vi "Main.vi"(7 "sweep rate, /min":dbl=0.2, 8 "sweep to:":dbl=4.0, 9 "sweep":T8(radio)=enum."2636a_smub") -> ()   [LabVIEW 2021] (continued)
                    n4073 = Number To Decimal String(number=w5385) -> (decimal integer string=w5387:string)  [unwired: 1 in]
                    n4074 = GPIB Write(0:w5387, 1:w5389, 2:i16 1 ("mode (0)")) -> ()  [unwired: 2 in, 2 out]
                  }
                  frame "2636_smua_step" {
                    # "sweep voltage on 2636a smua"
                    n4075 = property on="Step Channel" class="DigNum (strict)"() -> ("Value"=w5395:dbl)  [unwired: 2 in, 2 out]
                    n4076 = property on="Mini steps" class="DigNum (strict)"() -> ("Value"=w5393:dbl)  [unwired: 2 in, 2 out]
                    n4077 = property on="2614A_addr_step" class="VISAName"() -> ("Value"=w5394:refnum<visa-resource-name>)  [unwired: 2 in, 2 out]
                    n4078 = Subtract(x=w5392, y=w5395) -> (x-y=w5396:dbl)
                    n4079 = Divide(x=w5396, y=w5393) -> (x/y=w5397:dbl)
                    n4080 = for {
                      N: w5393 -> [_]
                      tunnel: w5395 -> [w5411]
                      tunnel: w5397 -> [w5410]
                      tunnel: w5394 -> [w5407]
                      i -> [w5406]
                      n4081 = Increment(x=w5406) -> (x+1=w5405:i32)
                      n4082 = Multiply(x=w5410, y=w5405) -> (x*y=w5409:dbl)
                      n4083 = Add(x=w5409, y=w5411) -> (x+y=w5403:dbl)
                      n4084 = property on="Lead Chanl_step" class="Enum (strict)"() -> ("Value"=w5402:T4)  [unwired: 2 in, 2 out]
                      n4085 = property on="step" class="RadioBtnsControl (strict)"() -> ("Value"=w5401:T5)  [unwired: 2 in, 2 out]
                      n4086 = call "setLevel.vi"("VISA resource name 2"=w5407, "Source"=Source."Voltage", "Channel"=Channel."a", "SourceLevel"=w5403) -> ("VISA resource name"=w5404:refnum<visa-resource-name>)  [unwired: 1 in, 2 out]
                      n4087 = property on="diagonal step" class="Bool (strict)"() -> ("Value"=w5400:bool)  [unwired: 2 in, 2 out]
                      n4088 = Wait (ms)(milliseconds to wait=u32 12) -> ()  [unwired: 1 out]
                      n4089 = Equal?(x=w5402, y=w5401) -> (x = y?=w5399:bool)
                      n4090 = property on="Current Step Value" class="DigNum (strict)"("Value"=w5403) -> ()  [unwired: 2 in, 2 out]
                      n4091 = And(x=w5400, y=w5399) -> (x .and. y?=w5398:bool)
                      n4092 = case shown="True" w5398 {
                        tunnel: w5403 -> [_ w5421]
                        tunnel: w5404 -> [_ w5416]
                        frame False {
                        }
                        frame True {
                          n4093 = property on="Step Slope" class="DigNum (strict)"() -> ("Value"=w5415:dbl)  [unwired: 2 in, 2 out]
                          n4094 = property on="Step Offset" class="DigNum (strict)"() -> ("Value"=w5414:dbl)  [unwired: 2 in, 2 out]
                          n4095 = Multiply(x=w5421, y=w5415) -> (x*y=w5420:dbl)
                          n4096 = Add(x=w5420, y=w5414) -> (x+y=w5417:dbl)
                          n4097 = call "setLevel.vi"("VISA resource name 2"=w5416, "Source"=Source."Voltage", "Channel"=Channel."b", "SourceLevel"=w5417) -> ()  [unwired: 1 in, 3 out]
                        }
                      }
                    }
                  }
                  frame "2636_smub_step" {
                    # "sweep voltage on 2636a smua"
                    n4098 = property on="Step Channel" class="DigNum (strict)"() -> ("Value"=w5425:dbl)  [unwired: 2 in, 2 out]
                    n4099 = property on="Mini steps" class="DigNum (strict)"() -> ("Value"=w5423:dbl)  [unwired: 2 in, 2 out]
                    n4100 = property on="2614A_addr_step" class="VISAName"() -> ("Value"=w5424:refnum<visa-resource-name>)  [unwired: 2 in, 2 out]
                    n4101 = Subtract(x=w5422, y=w5425) -> (x-y=w5426:dbl)
                    n4102 = Divide(x=w5426, y=w5423) -> (x/y=w5427:dbl)
                    n4103 = for {
                      N: w5423 -> [_]
                      tunnel: w5425 -> [w5441]
                      tunnel: w5427 -> [w5440]
                      tunnel: w5424 -> [w5437]
                      i -> [w5436]
                      n4104 = Increment(x=w5436) -> (x+1=w5435:i32)
                      n4105 = Multiply(x=w5440, y=w5435) -> (x*y=w5439:dbl)
                      n4106 = Add(x=w5439, y=w5441) -> (x+y=w5433:dbl)
                      n4107 = property on="Lead Chanl_step" class="Enum (strict)"() -> ("Value"=w5432:T4)  [unwired: 2 in, 2 out]
                      n4108 = property on="step" class="RadioBtnsControl (strict)"() -> ("Value"=w5431:T5)  [unwired: 2 in, 2 out]
                      n4109 = call "setLevel.vi"("VISA resource name 2"=w5437, "Source"=Source."Voltage", "Channel"=Channel."b", "SourceLevel"=w5433) -> ("VISA resource name"=w5434:refnum<visa-resource-name>)  [unwired: 1 in, 2 out]
                      n4110 = property on="diagonal step" class="Bool (strict)"() -> ("Value"=w5430:bool)  [unwired: 2 in, 2 out]
                      n4111 = Wait (ms)(milliseconds to wait=u32 12) -> ()  [unwired: 1 out]
                      n4112 = Equal?(x=w5432, y=w5431) -> (x = y?=w5429:bool)
                      n4113 = And(x=w5430, y=w5429) -> (x .and. y?=w5428:bool)
                      n4114 = property on="Current Step Value" class="DigNum (strict)"("Value"=w5433) -> ()  [unwired: 2 in, 2 out]
                      n4115 = case shown="True" w5428 {
                        tunnel: w5433 -> [_ w5451]
                        tunnel: w5434 -> [_ w5446]
                        frame False {
                        }
                        frame True {
                          n4116 = property on="Step Slope" class="DigNum (strict)"() -> ("Value"=w5445:dbl)  [unwired: 2 in, 2 out]
                          n4117 = property on="Step Offset" class="DigNum (strict)"() -> ("Value"=w5444:dbl)  [unwired: 2 in, 2 out]
                          n4118 = Multiply(x=w5451, y=w5445) -> (x*y=w5450:dbl)
                          n4119 = Add(x=w5450, y=w5444) -> (x+y=w5447:dbl)
                          n4120 = call "setLevel.vi"("VISA resource name 2"=w5446, "Source"=Source."Voltage", "Channel"=Channel."a", "SourceLevel"=w5447) -> ()  [unwired: 1 in, 3 out]
                        }
                      }
                    }
                  }
                  frame "time_step", Default {
                    # "do not sweep, just time"
                  }
                  frame "iPS_step" {
                    # "step magnetic field"
                    n4121 = stacked-sequence {
                      tunnel: w5452 -> [w5453 w5466 _]
                      frame #0 {
                        n4122 = property on="Table Index" class="DigNum (strict)"() -> ("Value"=w5456:dbl)  [unwired: 2 in, 2 out]
                        n4123 = Equal?(x=w5456, y=0.0) -> (x = y?=w5454:bool)
                        n4124 = case shown="False" w5454 {
                          tunnel: w5453 -> [w5457 w5459]
                          frame False {
                            n4125 = property on="FieldRate(T/min)" class="DigNum (strict)"() -> ("Value"=w5458:dbl)  [unwired: 2 in, 2 out]
                            n4126 = call "TRITON_Set field and rate.vi"("target field"=w5457, "Sweep rate"=w5458) -> ()  [unwired: 1 in, 1 out]
                          }
                          frame True {
                            n4127 = property on="FieldRate(T/min)" class="DigNum (strict)"() -> ("Value"=w5460:dbl)  [unwired: 2 in, 2 out]
                            n4128 = call "TRITON_Set field and rate.vi"("target field"=w5459, "Sweep rate"=w5460) -> ()  [unwired: 1 in, 1 out]
                          }
                        }
                      }
                      frame #1 {
                        n4129 = while {
                          tunnel: w5466 -> [w5494]
                          stop <- w5490 stop-if-true
                          n4130 = call "TRITON_Read Field.vi"() -> ("Measurement"=w5489:dbl)  [unwired: 2 in, 1 out]
                          n4131 = property on="Tolerance_Step" class="DigNum (strict)"() -> ("Value"=w5491:dbl)  [unwired: 2 in, 2 out]
                          n4132 = Subtract(x=w5489, y=w5494) -> (x-y=w5493:dbl)
                          n4133 = Wait (ms)(milliseconds to wait=u32 500) -> ()  [unwired: 1 out]
                          n4134 = Absolute Value(x=w5493) -> (abs(x)=w5492:dbl)
                          n4135 = Less Or Equal?(x=w5492, y=w5491) -> (x <= y?=w5490:bool)
                          n4136 = property on="Step Channel" class="DigNum (strict)"("Value"=w5489) -> ()  [unwired: 2 in, 2 out]
                          n4137 = property on="at field" class="Bool (strict)"("Value"=w5490) -> ()  [unwired: 2 in, 2 out]
                        }
                        n4138 = property on="Lead Chanl_step" class="Enum (strict)"() -> ("Value"=w5465:T4)  [unwired: 2 in, 2 out]
                        n4139 = property on="step" class="RadioBtnsControl (strict)"() -> ("Value"=w5464:T5)  [unwired: 2 in, 2 out]
                        n4140 = property on="diagonal step" class="Bool (strict)"() -> ("Value"=w5463:bool)  [unwired: 2 in, 2 out]
                        n4141 = Equal?(x=w5465, y=w5464) -> (x = y?=w5462:bool)
                        n4142 = And(x=w5463, y=w5462) -> (x .and. y?=w5461:bool)
                        n4143 = case shown="True" w5461 {
                          tunnel: w5466 -> [_ w5471]
                          frame False {
                          }
                          frame True {
                            n4144 = property on="Channel" class="Enum (strict)"() -> ("Value"=w5469:T3)  [unwired: 2 in, 2 out]
                            n4145 = property on="2614A_addr_step" class="VISAName"() -> ("Value"=w5470:refnum<visa-resource-name>)  [unwired: 2 in, 2 out]
                            n4146 = property on="Step Offset" class="DigNum (strict)"() -> ("Value"=w5476:dbl)  [unwired: 2 in, 2 out]
                            n4147 = property on="Step Slope" class="DigNum (strict)"() -> ("Value"=w5477:dbl)  [unwired: 2 in, 2 out]
                            n4148 = call "SinglePointMeasurement.vi"("Measure"=Measure."Voltage", "Channel"=w5469, "VISA resource name 2"=w5470) -> ("Measuremet"=w5467:dbl)  [unwired: 3 in, 4 out]
                            n4149 = Multiply(x=w5471, y=w5477) -> (x*y=w5478:dbl)
                            n4150 = Add(x=w5478, y=w5476) -> (x+y=w5472:dbl)
                            n4151 = Subtract(x=w5472, y=w5467) -> (x-y=w5474:dbl)
                            n4152 = property on="Mini steps" class="DigNum (strict)"() -> ("Value"=w5473:dbl)  [unwired: 2 in, 2 out]
                            n4153 = Divide(x=w5474, y=w5473) -> (x/y=w5475:dbl)
                            n4154 = for {
                              N: w5473 -> [_]
                              tunnel: w5475 -> [w5487]
                              tunnel: w5470 -> [w5484]
                              tunnel: w5467 -> [w5480]
                              i -> [w5482]
                              n4155 = Increment(x=w5482) -> (x+1=w5481:i32)
                              n4156 = Multiply(x=w5487, y=w5481) -> (x*y=w5486:dbl)
                              n4157 = Add(x=w5486, y=w5480) -> (x+y=w5483:dbl)
                              n4158 = property on="Channel" class="Enum (strict)"() -> ("Value"=w5479:T3)  [unwired: 2 in, 2 out]
                              n4159 = Wait (ms)(milliseconds to wait=u32 12) -> ()  [unwired: 1 out]
                              n4160 = call "setLevel.vi"("VISA resource name 2"=w5484, "Source"=Source."Voltage", "Channel"=w5479, "SourceLevel"=w5483) -> ()  [unwired: 1 in, 3 out]
                            }
                          }
                        }
                      }
                      frame #2 {
                        # "wait 5sec to stabilise the field"
                        n4161 = Wait (ms)(milliseconds to wait=u32 5000) -> ()  [unwired: 1 out]
                      }
                    }
                  }
                  frame "iTC_step" {
                    # "step temperature"
                    n4162 = stacked-sequence {
                      tunnel: w5497 -> [w5498 _ w5505]
                      frame #0 {
                        n4163 = Less Or Equal To 0?(x=w5498) -> (x <= 0?=w5502:bool)
                        n4164 = Select(t=0.0, s=w5502, f=w5498) -> (s? t:f=w5499:dbl)
                        n4165 = call "TRITON_Set Temperature.vi"("setpoint"=w5499) -> ()  [unwired: 2 in, 1 out]
                        n4166 = Wait (ms)(milliseconds to wait=u32 200) -> ()  [unwired: 1 out]
                      }
                      frame #1 {
                        n4167 = Wait (ms)(milliseconds to wait=u32 200) -> ()  [unwired: 1 out]
                      }
                      frame #2 {
                        n4168 = case shown="False" FALSE {
                          tunnel: w5505 -> [w5506 w5515]
                          frame True {
                            n4169 = while {
                              tunnel: w5506 -> [w5510]
                              stop <- w5512 stop-if-true
                              n4170 = Decrement(x=w5510) -> (x-1=w5509:dbl)
                              n4171 = call "TRITON_Read Temperature.vi"("Channel"="T_Channel") -> ("Measuremet"=w5508:dbl)  [unwired: 1 in, 1 out]
                              n4172 = Subtract(x=w5508, y=w5509) -> (x-y=w5514:dbl)
                              n4173 = property on="Step Channel" class="DigNum (strict)"("Value"=w5508) -> ()  [unwired: 2 in, 2 out]
                              n4174 = property on="Tolerance_Step" class="DigNum (strict)"() -> ("Value"=w5511:dbl)  [unwired: 2 in, 2 out]
                              n4175 = Absolute Value(x=w5514) -> (abs(x)=w5513:dbl)
                              n4176 = Less?(x=w5513, y=w5511) -> (x < y?=w5512:bool)
                              n4177 = property on="at field" class="Bool (strict)"("Value"=w5512) -> ()  [unwired: 2 in, 2 out]
                            }
                          }
                          frame False {
                            n4178 = while {
                              tunnel: w5515 -> [w5522]
                              stop <- w5519 stop-if-true
                              n4179 = property on="T_Channel" class="DigNum (strict)"() -> ("Value"=w5516:i32)  [unwired: 2 in, 2 out]
                              n4180 = call "TRITON_Read Temperature.vi"("Channel"=w5516) -> ("Measuremet"=w5517:dbl)  [unwired: 1 in, 1 out]
                              n4181 = property on="Tolerance_Step" class="DigNum (strict)"() -> ("Value"=w5518:dbl)  [unwired: 2 in, 2 out]
                              n4182 = Subtract(x=w5517, y=w5522) -> (x-y=w5521:dbl)
                              n4183 = property on="Step Channel" class="DigNum (strict)"("Value"=w5517) -> ()  [unwired: 2 in, 2 out]
                              n4184 = Absolute Value(x=w5521) -> (abs(x)=w5520:dbl)
                              n4185 = Less?(x=w5520, y=w5518) -> (x < y?=w5519:bool)
                              n4186 = property on="at field" class="Bool (strict)"("Value"=w5519) -> ()  [unwired: 2 in, 2 out]
                            }
                          }
                        }
                      }
                    }
                  }
                  frame "2461_Curr" {
                    n4187 = property on="2461_addr_step" class="VISAName"() -> ("Value"=w5523:refnum<visa-resource-name>)  [unwired: 2 in, 2 out]
                    n4188 = property on="Step Channel" class="DigNum (strict)"() -> ("Value"=w5526:dbl)  [unwired: 2 in, 2 out]
                    n4189 = property on="Mini steps" class="DigNum (strict)"() -> ("Value"=w5525:dbl)  [unwired: 2 in, 2 out]
                    n4190 = Subtract(x=w5524, y=w5526) -> (x-y=w5527:dbl)
                    n4191 = Divide(x=w5527, y=w5525) -> (x/y=w5528:dbl)
                    n4192 = for {
                      N: w5525 -> [_]
                      tunnel: w5526 -> [w5537]
                      tunnel: w5528 -> [w5536]
                      tunnel: w5523 -> [w5531]
                      i -> [w5533]
                      w5530 = u16 1 items=["Volts", "Current"] ("Function (0: Volts)")
                      n4193 = Increment(x=w5533) -> (x+1=w5532:i32)
                      n4194 = Multiply(x=w5536, y=w5532) -> (x*y=w5535:dbl)
                      n4195 = Add(x=w5535, y=w5537) -> (x+y=w5529:dbl)
                      n4196 = call <instrlib>:"Configure Source Level.vi"("Source Level (1.0)"=w5529, "Function (0: Volts)"=w5530, "VISA resource name"=w5531) -> ()  [unwired: 7 in, 2 out]
                      n4197 = Wait (ms)(milliseconds to wait=u32 12) -> ()  [unwired: 1 out]
                      n4198 = property on="Current Step Value" class="DigNum (strict)"("Value"=w5529) -> ()  [unwired: 2 in, 2 out]
                    }
                  }
                }
              }
              frame #1 {
                n4199 = property on="Current Step Value" class="DigNum (strict)"() -> ("Value"=w5542:dbl)  [unwired: 2 in, 2 out]
                n4200 = property on="Change Sweep Range" class="Bool (strict)"() -> ("Value"=w5538:bool)  [unwired: 2 in, 2 out]
                n4201 = property on="Step Channel" class="DigNum (strict)"("Value"=w5542) -> ()  [unwired: 2 in, 2 out]
                n4202 = case shown="True" w5538 {
                  frame False {
                  }
                  frame True {
                    n4203 = property on="Table Index" class="DigNum (strict)"() -> ("Value"=w5543:dbl)  [unwired: 2 in, 2 out]
                    n4204 = property on="Down          Up" class="Tbl (strict)"() -> ("Value"=w5549:string[][])  [unwired: 2 in, 2 out]
                    n4205 = Index Array(array=w5549, index (row)=w5543, index (col)=0 ("disabled index (col)")) -> (element=w5547:string)
                    n4206 = Index Array(array=w5549, index (row)=w5543, index (col)=1 ("disabled index (col)")) -> (element=w5544:string)
                    n4207 = Fract/Exp String To Number(string=w5547) -> (number=w5546:dbl)  [unwired: 3 in, 1 out]
                    n4208 = Fract/Exp String To Number(string=w5544) -> (number=w5545:dbl)  [unwired: 3 in, 1 out]
                    n4209 = property on="lower limit" class="DigNum (strict)"("Value"=w5546) -> ()  [unwired: 2 in, 2 out]
                    n4210 = property on="upper limit" class="DigNum (strict)"("Value"=w5545) -> ()  [unwired: 2 in, 2 out]
                  }
                }
                n4211 = property on="Wait Between Step(s)" class="DigNum (strict)"() -> ("Value"=w5541:i32)  [unwired: 2 in, 2 out]
                n4212 = Multiply(x=w5541, y=1000) -> (x*y=w5539:i32)
                n4213 = Wait (ms)(milliseconds to wait=w5539) -> ()  [unwired: 1 out]
              }
              frame #2 {
                n4214 = property on="Sweep Direction" class="Str"() -> ("Value"=w5551:string)  [unwired: 2 in, 2 out]
                n4215 = case shown="\"Ramp Down\", Default" w5551 {
                  frame "Sweep Down" {
                    n4216 = property on="Up Rate" class="DigNum (strict)" props=["Value"]() -> ()  [unwired: 2 in, 3 out]
                    n4217 = property on="upper limit" class="DigNum (strict)" props=["Value"]() -> ()  [unwired: 2 in, 3 out]
                    n4218 = property on="Down Rate" class="DigNum (strict)"() -> ("Value"=w5552:dbl)  [unwired: 2 in, 2 out]
                    n4219 = property on="lower limit" class="DigNum (strict)"() -> ("Value"=w5553:dbl)  [unwired: 2 in, 2 out]
                    n4220 = property on="sweep to:" class="DigNum (strict)"("Value"=w5553) -> ()  [unwired: 2 in, 2 out]
                    n4221 = property on="sweep rate, /min" class="DigNum (strict)"("Value"=w5552) -> ()  [unwired: 2 in, 2 out]
                  }
                  frame "Ramp Down", Default {
                    n4222 = property on="Down Rate" class="DigNum (strict)"() -> ("Value"=w5554:dbl)  [unwired: 2 in, 2 out]
                    n4223 = property on="lower limit" class="DigNum (strict)"() -> ("Value"=w5555:dbl)  [unwired: 2 in, 2 out]
                    n4224 = property on="sweep to:" class="DigNum (strict)"("Value"=w5555) -> ()  [unwired: 2 in, 2 out]
                    n4225 = property on="sweep rate, /min" class="DigNum (strict)"("Value"=w5554) -> ()  [unwired: 2 in, 2 out]
                  }
                  frame "Sweep Up" {
                    n4226 = property on="Up Rate" class="DigNum (strict)"() -> ("Value"=w5556:dbl)  [unwired: 2 in, 2 out]
                    n4227 = property on="upper limit" class="DigNum (strict)"() -> ("Value"=w5557:dbl)  [unwired: 2 in, 2 out]
                    n4228 = property on="sweep to:" class="DigNum (strict)"("Value"=w5557) -> ()  [unwired: 2 in, 2 out]
                    n4229 = property on="sweep rate, /min" class="DigNum (strict)"("Value"=w5556) -> ()  [unwired: 2 in, 2 out]
                  }
                  frame "True" {
                  }
                }
              }
              frame #3 {
                n4230 = Enqueue Element(queue=w5559, element="Start Sweep") -> ()  [unwired: 2 in, 3 out]
              }
            }
          }
          frame True {
            # "When step values are all finished"
            n4231 = property on="HyperLoop" class="Bool (strict)"() -> ("Value"=w5560:bool)  [unwired: 2 in, 2 out]
            n4232 = case shown="True" w5560 {
              tunnel: w5561 -> [w5567 w5572]
              frame False {
                n4233 = Enqueue Element(queue=w5567, element="Idle") -> ()  [unwired: 2 in, 3 out]
                n4234 = property on="Start Mapping" class="Bool"("DisabledEnum"=T10."Enabled" ("Disabled")) -> ()  [unwired: 2 in, 2 out]
                n4235 = property on="Stop Mapping" class="Bool"("DisabledEnum"=T10."Disabled and Grayed Out" ("Disabled")) -> ()  [unwired: 2 in, 2 out]
                n4236 = property on="Sweep Direction" class="Str"("Value"="Finished!" ("Sweep Direction"), "Text.TextColor"=u32 16711680 ("Text.Text Colors:Text Color")) -> ()  [unwired: 2 in, 2 out]
              }
              frame True {
                n4237 = Enqueue Element(queue=w5572, element="Step to Next HyperLoop Value") -> ()  [unwired: 2 in, 3 out]
                n4238 = property on="HyperLoop Index" class="DigNum (strict)"() -> ("Value"=w5570:dbl)  [unwired: 2 in, 2 out]
                n4239 = property on="Start Mapping" class="Bool"("DisabledEnum"=T10."Enabled" ("Disabled")) -> ()  [unwired: 2 in, 2 out]
                n4240 = property on="Stop Mapping" class="Bool"("DisabledEnum"=T10."Disabled and Grayed Out" ("Disabled")) -> ()  [unwired: 2 in, 2 out]
                n4241 = Increment(x=w5570) -> (x+1=w5571:dbl)
                n4242 = property on="HyperLoop Index" class="DigNum (strict)"("Value"=w5571) -> ()  [unwired: 2 in, 2 out]
                n4243 = property on="Sweep Direction" class="Str"("Value"="Finished!" ("Sweep Direction"), "Text.TextColor"=u32 16711680 ("Text.Text Colors:Text Color")) -> ()  [unwired: 2 in, 2 out]
              }
            }
          }
        }
      }
      frame "Step to Next HyperLoop Value" {
        n4244 = property on="HyperLoop Index" class="DigNum (strict)"() -> ("Value"=w5577:dbl)  [unwired: 2 in, 2 out]
        n4245 = property on="HyperLoop Steps" class="Tbl (strict)"() -> ("Value"=w5576:string[][])  [unwired: 2 in, 2 out]
        n4246 = Equal?(x=w5577, y=0) -> (x = y?=w5588:bool)
        n4247 = case shown="True" w5588 {
          tunnel: w5577 -> [w5596 w5602]
          tunnel: cluster{"Row":i32, "Column":i32} {"Row"=0, "Column"=0} ("Active Cell:Active Cell") -> [w5595 w5601]
          frame False {
            w5597 = 0 ("Column")
            n4248 = Decrement(x=w5596) -> (x-1=w5598:dbl)
            n4249 = Bundle By Name(cluster=w5595, "Row"=w5596, "Column"=w5597) -> (w5594:cluster{"Row":i32, "Column":i32})
            n4250 = Bundle By Name(cluster=w5594, "Row"=w5598, "Column"=w5597) -> (w5592:cluster{"Row":i32, "Column":i32})
            n4251 = property on="HyperLoop Steps" class="Tbl (strict)"("Active Cell"=w5592, "Cell BG Color"=u32 16711680 ("Active Cell:Cell Background Color")) -> ()  [unwired: 2 in, 2 out]
            n4252 = property on="HyperLoop Steps" class="Tbl (strict)"("Active Cell"=w5594, "Cell BG Color"=u32 16776072 ("Active Cell:Cell Background Color")) -> ()  [unwired: 2 in, 2 out]
          }
          frame True {
            n4253 = Bundle By Name(cluster=w5601, "Row"=w5602, "Column"=0) -> (w5600:cluster{"Row":i32, "Column":i32})
            n4254 = property on="HyperLoop Steps" class="Tbl (strict)"("Active Cell"=w5600, "Cell BG Color"=u32 16776072 ("Active Cell:Cell Background Color")) -> ()  [unwired: 2 in, 2 out]
          }
        }
        n4255 = call <vilib>:"Space Constant.vi"() -> ("String"=w5586:string)
        n4256 = Index Array(array=w5576, index (row)=w5577, index (col)=0 ("disabled index (col)")) -> (element=w5585:string)
        n4257 = call <vilib>:"Search and Replace Pattern.vi"("string"=w5585, "regular expression (\"\")"=w5586, "replace string (\"\")"="" ("replace string (\"\")"), "replace all? (F)"=TRUE) -> ("result string"=w5589:string)  [unwired: 1 in, 1 out]
        n4258 = Equal?(x="", y=w5589) -> (x = y?=w5587:bool)
        n4259 = Fract/Exp String To Number(string=w5589) -> (number=w5590:dbl)  [unwired: 3 in, 1 out]
        n4260 = case shown="False" w5587 {
          tunnel: w5590 -> [w5604 _]
          tunnel: w5579 -> [w5605 w5781]
          frame False {
            # "When step values are not finished"
            n4261 = stacked-sequence {
              tunnel: w5604 -> [w5607 _ _]
              tunnel: w5605 -> [_ _ _]
              frame #0 {
                # "1 = 2400 1\n2 = 2400 2\n\n4 = 2636a smua\n5 = 2636a smub\n6 = do not sweep, just time\n7 = iPS, magnetic field \n8 = iTC, temperature"
                # "set next value in the sweep"
                n4262 = property on="step_hyper" class="RadioBtnsControl (strict)"() -> ("Value"=w5606:T6)  [unwired: 2 in, 2 out]
                n4263 = case shown="\"iTC_HyperLoop\"" w5606 {
                  tunnel: w5607 -> [w5609 w5616 _ _ _ w5674 w5738]
                  tunnel: w5607 -> [_ _ w5625 w5651 _ _ _]
                  frame "2400_1_HyperLoop" {
                    # "sweep voltage on 2400 1"
                    n4264 = property on="2400_1_addr_hyper" class="DigNum (strict)"() -> ("Value"=w5608:u8)  [unwired: 2 in, 2 out]
                    n4265 = Number To Fractional String(number=w5609) -> (F-format string=w5614:string)  [unwired: 3 in]
                    n4266 = Concatenate Strings(":INIT:IMM; :SOUR:VOLT:LEV:IMM:AMPL " ("data"), w5614) -> (w5612:string)
                    n4267 = Number To Decimal String(number=w5608) -> (decimal integer string=w5610:string)  [unwired: 1 in]
                    n4268 = GPIB Write(0:w5610, 1:w5612, 2:i16 1 ("mode (0)")) -> ()  [unwired: 2 in, 2 out]
                  }
                  frame "2400_2_HyperLoop" {
                    # "sweep voltage on 2400 2"
                    n4269 = property on="2400_2_addr_hyper" class="DigNum (strict)"() -> ("Value"=w5615:u8)  [unwired: 2 in, 2 out]
                    n4270 = Number To Fractional String(number=w5616) -> (F-format string=w5621:string)  [unwired: 3 in]
                    n4271 = Concatenate Strings(":INIT:IMM; :SOUR:CURR:LEV:IMM:AMPL " ("data"), w5621) -> (w5619:string)
                    n4272 = Number To Decimal String(number=w5615) -> (decimal integer string=w5617:string)  [unwired: 1 in]
                    n4273 = GPIB Write(0:w5617, 1:w5619, 2:i16 1 ("mode (0)")) -> ()  [unwired: 2 in, 2 out]
                  }
                  frame "2636_smua_HyperLoop" {
                    # "sweep voltage on 2636a smua"
                    n4274 = property on="Hyper Channel" class="DigNum (strict)"() -> ("Value"=w5622:dbl)  [unwired: 2 in, 2 out]
                    n4275 = property on="2336A_addr_hyper" class="VISAName"() -> ("Value"=w5623:refnum<visa-resource-name>)  [unwired: 2 in, 2 out]
                    n4276 = property on="Hyper_Mini steps" class="DigNum (strict)"() -> ("Value"=w5624:dbl)  [unwired: 2 in, 2 out]
                    n4277 = Subtract(x=w5625, y=w5622) -> (x-y=w5626:dbl)
                    n4278 = Divide(x=w5626, y=w5624) -> (x/y=w5627:dbl)
                    n4279 = for {
                      N: w5624 -> [_]
                      tunnel: w5622 -> [w5637]
                      tunnel: w5627 -> [w5636]
                      tunnel: w5623 -> [w5633]
                      i -> [w5632]
                      n4280 = Increment(x=w5632) -> (x+1=w5631:i32)
                      n4281 = Multiply(x=w5636, y=w5631) -> (x*y=w5635:dbl)
                      n4282 = Add(x=w5635, y=w5637) -> (x+y=w5628:dbl)
                      n4283 = call "setLevel.vi"("VISA resource name 2"=w5633, "Source"=Source."Voltage", "Channel"=Channel."a", "SourceLevel"=w5628) -> ("VISA resource name"=w5630:refnum<visa-resource-name>)  [unwired: 1 in, 2 out]
                      n4284 = Wait (ms)(milliseconds to wait=u32 12) -> ()  [unwired: 1 out]
                      n4285 = property on="diagonal_hyper" class="Bool (strict)"() -> ("Value"=w5629:bool)  [unwired: 2 in, 2 out]
                      n4286 = property on="Hyper Channel" class="DigNum (strict)"("Value"=w5628) -> ()  [unwired: 2 in, 2 out]
                      n4287 = case shown="True" w5629 {
                        tunnel: w5628 -> [_ w5647]
                        tunnel: w5630 -> [_ w5642]
                        frame False {
                        }
                        frame True {
                          n4288 = property on="Hyper Offset" class="DigNum (strict)"() -> ("Value"=w5640:dbl)  [unwired: 2 in, 2 out]
                          n4289 = property on="Hyper Slope" class="DigNum (strict)"() -> ("Value"=w5641:dbl)  [unwired: 2 in, 2 out]
                          n4290 = Multiply(x=w5647, y=w5641) -> (x*y=w5646:dbl)
                          n4291 = Add(x=w5646, y=w5640) -> (x+y=w5643:dbl)
                          n4292 = call "setLevel.vi"("VISA resource name 2"=w5642, "Source"=Source."Voltage", "Channel"=Channel."b", "SourceLevel"=w5643) -> ()  [unwired: 1 in, 3 out]
                        }
                      }
                    }
                  }
                  frame "2636_smub_HyperLoop" {
                    # "sweep voltage on 2636a smua"
                    n4293 = property on="Hyper Channel" class="DigNum (strict)"() -> ("Value"=w5648:dbl)  [unwired: 2 in, 2 out]
                    n4294 = property on="Hyper_Mini steps" class="DigNum (strict)"() -> ("Value"=w5650:dbl)  [unwired: 2 in, 2 out]
                    n4295 = property on="2336A_addr_hyper" class="VISAName"() -> ("Value"=w5649:refnum<visa-resource-name>)  [unwired: 2 in, 2 out]
                    n4296 = Subtract(x=w5651, y=w5648) -> (x-y=w5652:dbl)
                    n4297 = Divide(x=w5652, y=w5650) -> (x/y=w5653:dbl)
                    n4298 = for {
                      N: w5650 -> [_]
                      tunnel: w5648 -> [w5663]
                      tunnel: w5653 -> [w5662]
                      tunnel: w5649 -> [w5659]
                      i -> [w5658]
                      n4299 = Increment(x=w5658) -> (x+1=w5657:i32)
                      n4300 = Multiply(x=w5662, y=w5657) -> (x*y=w5661:dbl)
                      n4301 = Add(x=w5661, y=w5663) -> (x+y=w5654:dbl)
                      n4302 = property on="diagonal_hyper" class="Bool (strict)"() -> ("Value"=w5655:bool)  [unwired: 2 in, 2 out]
                      n4303 = call "setLevel.vi"("VISA resource name 2"=w5659, "Source"=Source."Voltage", "Channel"=Channel."b", "SourceLevel"=w5654) -> ("VISA resource name"=w5656:refnum<visa-resource-name>)  [unwired: 1 in, 2 out]
                      n4304 = Wait (ms)(milliseconds to wait=u32 12) -> ()  [unwired: 1 out]
                      n4305 = case shown="True" w5655 {
                        tunnel: w5654 -> [_ w5673]
                        tunnel: w5656 -> [_ w5668]
                        frame False {
                        }
                        frame True {
                          n4306 = property on="Hyper Offset" class="DigNum (strict)"() -> ("Value"=w5666:dbl)  [unwired: 2 in, 2 out]
                          n4307 = property on="Hyper Slope" class="DigNum (strict)"() -> ("Value"=w5667:dbl)  [unwired: 2 in, 2 out]
                          n4308 = Multiply(x=w5673, y=w5667) -> (x*y=w5672:dbl)
                          n4309 = Add(x=w5672, y=w5666) -> (x+y=w5669:dbl)
                          n4310 = call "setLevel.vi"("VISA resource name 2"=w5668, "Source"=Source."Voltage", "Channel"=Channel."a", "SourceLevel"=w5669) -> ()  [unwired: 1 in, 3 out]
                        }
                      }
                      n4311 = property on="Hyper Channel" class="DigNum (strict)"("Value"=w5654) -> ()  [unwired: 2 in, 2 out]
                    }
                  }
                  frame "time_HyperLoop", Default {
                    # "do not sweep, just time"
                  }
                  frame "iPS_HyperLoop" {
                    # "step magnetic field"
                    n4312 = stacked-sequence {
                      tunnel: w5674 -> [_ _ _ _ w5689 _ _ _ w5701 _ w5704 _]
                      frame #0 {
                        n4313 = property on="HyperLoop Index" class="DigNum (strict)"() -> ("Value"=w5675:dbl)  [unwired: 2 in, 2 out]
                        n4314 = Equal?(x=w5675, y=0.0) -> (x = y?=w5676:bool)
                        n4315 = case shown="True" w5676 {
                          frame False {
                          }
                          frame True {
                            n4316 = property on="iPS _addr_hyper" class="VISAName"() -> ("Value"=w5680:refnum<visa-resource-name>)  [unwired: 2 in, 2 out]
                            n4317 = property on="Hyper_FieldRate\n(T/min)" class="DigNum (strict)"() -> ("Value"=w5678:dbl)  [unwired: 2 in, 2 out]
                            n4318 = call "iPSset.vi"("Field Rate, T/min"=w5678, "iPSSetCtrl"=iPSsetCtrl."Set Target Field Rate", "VISA resource name"=w5680) -> ("VISA resource name out"=w5679:refnum<visa-resource-name>)  [unwired: 5 in, 3 out]
                            n4319 = property on="iPS _addr_hyper" class="VISAName"("Value"=w5679) -> ()  [unwired: 2 in, 2 out]
                          }
                        }
                      }
                      frame #1 {
                        n4320 = Wait (ms)(milliseconds to wait=u32 500) -> ()  [unwired: 1 out]
                      }
                      frame #2 {
                        n4321 = property on="iPS _addr_hyper" class="VISAName"() -> ("Value"=w5683:refnum<visa-resource-name>)  [unwired: 2 in, 2 out]
                        n4322 = call "iPSset.vi"("iPSSetCtrl"=iPSsetCtrl."Hold", "VISA resource name"=w5683) -> ("VISA resource name out"=w5684:refnum<visa-resource-name>)  [unwired: 6 in, 3 out]
                        n4323 = property on="iPS _addr_hyper" class="VISAName"("Value"=w5684) -> ()  [unwired: 2 in, 2 out]
                      }
                      frame #3 {
                        n4324 = Wait (ms)(milliseconds to wait=u32 500) -> ()  [unwired: 1 out]
                      }
                      frame #4 {
                        n4325 = property on="iPS _addr_hyper" class="VISAName"() -> ("Value"=w5687:refnum<visa-resource-name>)  [unwired: 2 in, 2 out]
                        n4326 = call "iPSset.vi"("Target Field, T"=w5689, "iPSSetCtrl"=iPSsetCtrl."Set Target Field", "VISA resource name"=w5687) -> ("VISA resource name out"=w5688:refnum<visa-resource-name>)  [unwired: 5 in, 3 out]
                        n4327 = property on="iPS _addr_hyper" class="VISAName"("Value"=w5688) -> ()  [unwired: 2 in, 2 out]
                      }
                      frame #5 {
                        n4328 = Wait (ms)(milliseconds to wait=u32 500) -> ()  [unwired: 1 out]
                      }
                      frame #6 {
                        n4329 = property on="iPS _addr_hyper" class="VISAName"() -> ("Value"=w5692:refnum<visa-resource-name>)  [unwired: 2 in, 2 out]
                        n4330 = call "iPSset.vi"("iPSSetCtrl"=iPSsetCtrl."Hold", "VISA resource name"=w5692) -> ("VISA resource name out"=w5693:refnum<visa-resource-name>)  [unwired: 6 in, 3 out]
                        n4331 = property on="iPS _addr_hyper" class="VISAName"("Value"=w5693) -> ()  [unwired: 2 in, 2 out]
                      }
                      frame #7 {
                        n4332 = Wait (ms)(milliseconds to wait=u32 500) -> ()  [unwired: 1 out]
                      }
                      frame #8 {
                        n4333 = Equal To 0?(x=w5701) -> (x = 0?=w5700:bool)
                        n4334 = property on="iPS _addr_hyper" class="VISAName"() -> ("Value"=w5696:refnum<visa-resource-name>)  [unwired: 2 in, 2 out]
                        n4335 = Select(t=iPSsetCtrl."Go to Zero" ("iPSSetCtrl"), s=w5700, f=iPSsetCtrl."Go to Field" ("iPSSetCtrl")) -> (s? t:f=w5697:T16)
                        n4336 = call "iPSset.vi"("iPSSetCtrl"=w5697, "VISA resource name"=w5696) -> ()  [unwired: 6 in, 4 out]
                      }
                      frame #9 {
                        n4337 = Wait (ms)(milliseconds to wait=u32 500) -> ()  [unwired: 1 out]
                      }
                      frame #10 {
                        n4338 = while {
                          tunnel: w5704 -> [w5735]
                          stop <- w5731 stop-if-true
                          n4339 = property on="iPS _addr_hyper" class="VISAName"() -> ("Value"=w5730:refnum<visa-resource-name>)  [unwired: 2 in, 2 out]
                          n4340 = call "iPSread.vi"("iPSreadCtrl"=iPSreadCtrl."MagnetField", "VISA resource name"=w5730) -> ("number"=w5727:dbl, "VISA resource name out"=w5729:refnum<visa-resource-name>)  [unwired: 6 in, 2 out]
                          n4341 = property on="Tolerance_Hyper" class="DigNum (strict)"() -> ("Value"=w5728:dbl)  [unwired: 2 in, 2 out]
                          n4342 = property on="iPS _addr_hyper" class="VISAName"("Value"=w5729) -> ()  [unwired: 2 in, 2 out]
                          n4343 = Wait (ms)(milliseconds to wait=u32 500) -> ()  [unwired: 1 out]
                          n4344 = Subtract(x=w5727, y=w5735) -> (x-y=w5734:dbl)
                          n4345 = Absolute Value(x=w5734) -> (abs(x)=w5733:dbl)
                          n4346 = Less Or Equal?(x=w5733, y=w5728) -> (x <= y?=w5731:bool)
                          n4347 = property on="Hyper Channel" class="DigNum (strict)"("Value"=w5727) -> ()  [unwired: 2 in, 2 out]
                          n4348 = property on="at field_hyper" class="Bool (strict)"("Value"=w5731) -> ()  [unwired: 2 in, 2 out]
                        }
                        n4349 = property on="diagonal_hyper" class="Bool (strict)"() -> ("Value"=w5703:bool)  [unwired: 2 in, 2 out]
                        n4350 = case shown="True" w5703 {
                          tunnel: w5704 -> [_ w5712]
                          frame False {
                          }
                          frame True {
                            n4351 = property on="Channel hyper" class="Enum (strict)"() -> ("Value"=w5706:T3)  [unwired: 2 in, 2 out]
                            n4352 = property on="2336A_addr_hyper" class="VISAName"() -> ("Value"=w5705:refnum<visa-resource-name>)  [unwired: 2 in, 2 out]
                            n4353 = property on="Hyper Offset" class="DigNum (strict)"() -> ("Value"=w5708:dbl)  [unwired: 2 in, 2 out]
                            n4354 = property on="Hyper Slope" class="DigNum (strict)"() -> ("Value"=w5709:dbl)  [unwired: 2 in, 2 out]
                            n4355 = call "SinglePointMeasurement.vi"("Measure"=Measure."Voltage", "Channel"=w5706, "VISA resource name 2"=w5705) -> ("Measuremet"=w5710:dbl)  [unwired: 3 in, 4 out]
                            n4356 = Multiply(x=w5712, y=w5709) -> (x*y=w5716:dbl)
                            n4357 = property on="Hyper_Mini steps" class="DigNum (strict)"() -> ("Value"=w5707:dbl)  [unwired: 2 in, 2 out]
                            n4358 = Add(x=w5716, y=w5708) -> (x+y=w5713:dbl)
                            n4359 = Subtract(x=w5713, y=w5710) -> (x-y=w5714:dbl)
                            n4360 = Divide(x=w5714, y=w5707) -> (x/y=w5715:dbl)
                            n4361 = for {
                              N: w5707 -> [_]
                              tunnel: w5715 -> [w5725]
                              tunnel: w5705 -> [w5722]
                              tunnel: w5710 -> [w5718]
                              i -> [w5720]
                              n4362 = Increment(x=w5720) -> (x+1=w5719:i32)
                              n4363 = Multiply(x=w5725, y=w5719) -> (x*y=w5724:dbl)
                              n4364 = Add(x=w5724, y=w5718) -> (x+y=w5721:dbl)
                              n4365 = property on="Channel 2" class="Enum (strict)"() -> ("Value"=w5717:T3)  [unwired: 2 in, 2 out]
                              n4366 = Wait (ms)(milliseconds to wait=u32 12) -> ()  [unwired: 1 out]
                              n4367 = call "setLevel.vi"("VISA resource name 2"=w5722, "Source"=Source."Voltage", "Channel"=w5717, "SourceLevel"=w5721) -> ()  [unwired: 1 in, 3 out]
                            }
                          }
                        }
                      }
                      frame #11 {
                        n4368 = Wait (ms)(milliseconds to wait=u32 500) -> ()  [unwired: 1 out]
                      }
                    }
                  }
                  frame "iTC_HyperLoop" {
                    # "step temperature"
                    n4369 = stacked-sequence {
                      tunnel: w5738 -> [w5746 w5750 w5756]
                      frame #0 {
                        n4370 = property on="iTC_addr_hyper" class="VISAName"() -> ("Value"=w5740:refnum<visa-resource-name>)  [unwired: 2 in, 2 out]
                        n4371 = Decrement(x=w5746) -> (x-1=w5743:dbl)
                        n4372 = Less Or Equal To 0?(x=w5743) -> (x <= 0?=w5745:bool)
                        n4373 = Select(t=0.0, s=w5745, f=w5743) -> (s? t:f=w5742:dbl)
                        n4374 = call "iTCset.vi"("Set Point"=w5742, "iTCSetCtrl"=iTCsetCtrl."Set VTI Temp", "VISA resource name"=w5740) -> ("VISA resource name out"=w5739:refnum<visa-resource-name>)  [unwired: 5 in, 3 out]
                        n4375 = Wait (ms)(milliseconds to wait=u32 200) -> ()  [unwired: 1 out]
                        n4376 = property on="iTC_addr_hyper" class="VISAName"("Value"=w5739) -> ()  [unwired: 2 in, 2 out]
                      }
                      frame #1 {
                        n4377 = property on="iTC_addr_hyper" class="VISAName"() -> ("Value"=w5748:refnum<visa-resource-name>)  [unwired: 2 in, 2 out]
                        n4378 = Less Or Equal To 0?(x=w5750) -> (x <= 0?=w5754:bool)
                        n4379 = Select(t=0.0, s=w5754, f=w5750) -> (s? t:f=w5752:dbl)
                        n4380 = call "iTCset.vi"("Set Point"=w5752, "iTCSetCtrl"=iTCsetCtrl."Set Sample Temp", "VISA resource name"=w5748) -> ("VISA resource name out"=w5749:refnum<visa-resource-name>)  [unwired: 5 in, 3 out]
                        n4381 = property on="iTC_addr_hyper" class="VISAName"("Value"=w5749) -> ()  [unwired: 2 in, 2 out]
                        n4382 = Wait (ms)(milliseconds to wait=u32 200) -> ()  [unwired: 1 out]
                      }
                      frame #2 {
                        n4383 = while {
                          tunnel: w5756 -> [w5763]
                          stop <- w5759 stop-if-true
                          n4384 = property on="iTC_addr_hyper" class="VISAName"() -> ("Value"=w5760:refnum<visa-resource-name>)  [unwired: 2 in, 2 out]
                          n4385 = property on="Tolerance_Hyper" class="DigNum (strict)"() -> ("Value"=w5758:dbl)  [unwired: 2 in, 2 out]
                          n4386 = call "iTCread.vi"("VISA resource name"=w5760, "iTCreadCtrl"=iTCreadCtrl."Sample Temp") -> ("number"=w5757:dbl)  [unwired: 5 in, 3 out]
                          n4387 = Subtract(x=w5757, y=w5763) -> (x-y=w5762:dbl)
                          n4388 = Absolute Value(x=w5762) -> (abs(x)=w5761:dbl)
                          n4389 = property on="Hyper Channel" class="DigNum (strict)"("Value"=w5757) -> ()  [unwired: 2 in, 2 out]
                          n4390 = Less?(x=w5761, y=w5758) -> (x < y?=w5759:bool)
                          n4391 = property on="at field_hyper" class="Bool (strict)"("Value"=w5759) -> ()  [unwired: 2 in, 2 out]
                        }
                      }
                    }
                  }
                }
              }
              frame #1 {
                # "Set current hyper channel and wait expected time"
                n4392 = property on="Current Hyper Value" class="DigNum (strict)"() -> ("Value"=w5766:dbl)  [unwired: 2 in, 2 out]
                n4393 = property on="Wait Between Hyper" class="DigNum (strict)"() -> ("Value"=w5765:i32)  [unwired: 2 in, 2 out]
                n4394 = property on="Hyper Channel" class="DigNum (strict)"("Value"=w5766) -> ()  [unwired: 2 in, 2 out]
                n4395 = Multiply(x=w5765, y=1000) -> (x*y=w5767:i32)
                n4396 = Wait (ms)(milliseconds to wait=w5767) -> ()  [unwired: 1 out]
              }
              frame #2 {
                n4397 = stacked-sequence {
                  frame #0 {
                    # "Check if need to swap step direction"
                    n4398 = property on="SwapStepDirection" class="Bool (strict)"() -> ("Value"=w5769:bool)  [unwired: 2 in, 2 out]
                    n4399 = case shown="True" w5769 {
                      frame False {
                      }
                      frame True {
                        n4400 = stacked-sequence {
                          frame #0 {
                            n4401 = property on="HyperLoop Index" class="DigNum (strict)"() -> ("Value"=w5771:dbl)  [unwired: 2 in, 2 out]
                            n4402 = Equal To 0?(x=w5771) -> (x = 0?=w5770:bool)
                            n4403 = case shown="False" w5770 {
                              frame False {
                                n4404 = property on="to" class="DigNum (strict)"() -> ("Value"=w5775:dbl)  [unwired: 2 in, 2 out]
                                n4405 = property on="from" class="DigNum (strict)"() -> ("Value"=w5774:dbl)  [unwired: 2 in, 2 out]
                                n4406 = Swap Values(12:w5775, 14:w5774) -> (1:w5773:dbl, 3:w5772:dbl)  [unwired: 1 in]
                                n4407 = property on="from" class="DigNum (strict)"("Value"=w5772) -> ()  [unwired: 2 in, 2 out]
                                n4408 = property on="to" class="DigNum (strict)"("Value"=w5773) -> ()  [unwired: 2 in, 2 out]
                              }
                              frame True {
                              }
                            }
                          }
                          frame #1 {
                            n4409 = property on="HyperLoop Index" class="DigNum (strict)"() -> ("Value"=w5777:dbl)  [unwired: 2 in, 2 out]
                            n4410 = Equal To 0?(x=w5777) -> (x = 0?=w5776:bool)
                            n4411 = case shown="False" w5776 {
                              frame False {
                                n4412 = property on="Hidden_HyperLoop_Swap" class="Bool (strict)"() -> ("Value"=w5778:bool)  [unwired: 2 in, 2 out]
                                n4413 = property on="Hidden_HyperLoop_Swap" class="Bool (strict)"("Val(Sgnl)"=w5778) -> ()  [unwired: 2 in, 2 out]
                              }
                              frame True {
                              }
                            }
                          }
                        }
                      }
                    }
                  }
                  frame #1 {
                    # "Trigger \"start mapping\" event"
                    n4414 = property on="HyperLoop Hidden" class="Bool (strict)"() -> ("Value"=w5779:bool)  [unwired: 2 in, 2 out]
                    n4415 = property on="HyperLoop Hidden" class="Bool (strict)"("Val(Sgnl)"=w5779) -> ()  [unwired: 2 in, 2 out]
                  }
                }
              }
            }
            n4416 = property on="Current Hyper Value" class="DigNum (strict)"("Value"=w5604) -> ()  [unwired: 2 in, 2 out]
          }
          frame True {
            # "When step values are all finished"
            n4417 = property on="SuperHyper" class="Bool (strict)"() -> ("Value"=w5780:bool)  [unwired: 2 in, 2 out]
            n4418 = case shown="True" w5780 {
              tunnel: w5781 -> [w5787 w5795]
              frame False {
                n4419 = Enqueue Element(queue=w5787, element="Idle") -> ()  [unwired: 2 in, 3 out]
                n4420 = property on="Stop HyperLoop" class="Bool"("DisabledEnum"=T10."Disabled and Grayed Out" ("Disabled")) -> ()  [unwired: 2 in, 2 out]
                n4421 = property on="Start HyperLoop" class="Bool"("DisabledEnum"=T10."Enabled" ("Disabled")) -> ()  [unwired: 2 in, 2 out]
                n4422 = property on="Sweep Direction 2" class="Str"("Value"="Finished!" ("Sweep Direction"), "Text.TextColor"=u32 16711680 ("Text.Text Colors:Text Color")) -> ()  [unwired: 2 in, 2 out]
              }
              frame True {
                n4423 = Enqueue Element(queue=w5795, element="Step to Next SuperHyper Value") -> ()  [unwired: 2 in, 3 out]
                n4424 = property on="SuperHyper_Index" class="DigNum (strict)"() -> ("Value"=w5793:dbl)  [unwired: 2 in, 2 out]
                n4425 = Increment(x=w5793) -> (x+1=w5792:dbl)
                n4426 = property on="Start HyperLoop" class="Bool"("DisabledEnum"=T10."Enabled" ("Disabled")) -> ()  [unwired: 2 in, 2 out]
                n4427 = property on="Stop HyperLoop" class="Bool"("DisabledEnum"=T10."Disabled and Grayed Out" ("Disabled")) -> ()  [unwired: 2 in, 2 out]
                n4428 = property on="SuperHyper_Index" class="DigNum (strict)"("Value"=w5792) -> ()  [unwired: 2 in, 2 out]
                n4429 = property on="Sweep Direction_Hyper" class="Str"("Value"="Finished!" ("Sweep Direction"), "Text.TextColor"=u32 16711680 ("Text.Text Colors:Text Color")) -> ()  [unwired: 2 in, 2 out]
              }
            }
          }
        }
      }
      frame "Step to Next SuperHyper Value" {
        n4430 = property on="SuperHyper_Index" class="DigNum (strict)"() -> ("Value"=w5796:dbl)  [unwired: 2 in, 2 out]
        n4431 = property on="SuperHyper Steps" class="Tbl (strict)"() -> ("Value"=w5797:string[][])  [unwired: 2 in, 2 out]
        n4432 = Equal?(x=w5796, y=0) -> (x = y?=w5808:bool)
        n4433 = case shown="False" w5808 {
          tunnel: w5796 -> [w5816 w5822]
          tunnel: cluster{"Row":i32, "Column":i32} {"Row"=0, "Column"=0} ("Active Cell:Active Cell") -> [w5815 w5821]
          frame False {
            w5817 = 0 ("Column")
            n4434 = Decrement(x=w5816) -> (x-1=w5818:dbl)
            n4435 = Bundle By Name(cluster=w5815, "Row"=w5816, "Column"=w5817) -> (w5814:cluster{"Row":i32, "Column":i32})
            n4436 = Bundle By Name(cluster=w5814, "Row"=w5818, "Column"=w5817) -> (w5812:cluster{"Row":i32, "Column":i32})
            n4437 = property on="SuperHyper Steps" class="Tbl (strict)"("Active Cell"=w5814, "Cell BG Color"=u32 16776072 ("Active Cell:Cell Background Color")) -> ()  [unwired: 2 in, 2 out]
            n4438 = property on="SuperHyper Steps" class="Tbl (strict)"("Active Cell"=w5812, "Cell BG Color"=u32 16711680 ("Active Cell:Cell Background Color")) -> ()  [unwired: 2 in, 2 out]
          }
          frame True {
            n4439 = Bundle By Name(cluster=w5821, "Row"=w5822, "Column"=0) -> (w5820:cluster{"Row":i32, "Column":i32})
            n4440 = property on="SuperHyper Steps" class="Tbl (strict)"("Active Cell"=w5820, "Cell BG Color"=u32 16776072 ("Active Cell:Cell Background Color")) -> ()  [unwired: 2 in, 2 out]
          }
        }
        n4441 = call <vilib>:"Space Constant.vi"() -> ("String"=w5806:string)
        n4442 = Index Array(array=w5797, index (row)=w5796, index (col)=0 ("disabled index (col)")) -> (element=w5805:string)
        n4443 = call <vilib>:"Search and Replace Pattern.vi"("string"=w5805, "regular expression (\"\")"=w5806, "replace string (\"\")"="" ("replace string (\"\")"), "replace all? (F)"=TRUE) -> ("result string"=w5809:string)  [unwired: 1 in, 1 out]
        n4444 = Equal?(x="", y=w5809) -> (x = y?=w5807:bool)
        n4445 = Fract/Exp String To Number(string=w5809) -> (number=w5810:dbl)  [unwired: 3 in, 1 out]
        n4446 = case shown="False" w5807 {
          tunnel: w5810 -> [w5824 _]
          tunnel: w5799 -> [w5825 w6003]
          frame False {
            # "When step values are not finished"
            n4447 = stacked-sequence {
              tunnel: w5824 -> [w5827 _ _ _]
              tunnel: w5825 -> [_ _ _ _]
              frame #0 {
                # "1 = 2400 1\n2 = 2400 2\n\n4 = 2636a smua\n5 = 2636a smub\n6 = do not sweep, just time\n7 = iPS, magnetic field \n8 = iTC, temperature"
                # "set next value in the sweep"
                n4448 = property on="step_super" class="RadioBtnsControl (strict)"() -> ("Value"=w5826:T7)  [unwired: 2 in, 2 out]
                n4449 = case shown="\"2636_smub_SuperHyper\"" w5826 {
                  tunnel: w5827 -> [w5829 w5836 _ _ _ w5894 w5958]
                  tunnel: w5827 -> [_ _ w5845 w5871 _ _ _]
                  frame "2400_1_SuperHyper" {
                    # "sweep voltage on 2400 1"
                    n4450 = property on="2400_1_addr_superhyper" class="DigNum (strict)"() -> ("Value"=w5828:u8)  [unwired: 2 in, 2 out]
                    n4451 = Number To Fractional String(number=w5829) -> (F-format string=w5834:string)  [unwired: 3 in]
                    n4452 = Concatenate Strings(":INIT:IMM; :SOUR:VOLT:LEV:IMM:AMPL " ("data"), w5834) -> (w5832:string)
                    n4453 = Number To Decimal String(number=w5828) -> (decimal integer string=w5830:string)  [unwired: 1 in]
                    n4454 = GPIB Write(0:w5830, 1:w5832, 2:i16 1 ("mode (0)")) -> ()  [unwired: 2 in, 2 out]
                  }
                  frame "2400_2_SuperHyper" {
                    # "sweep voltage on 2400 2"
                    n4455 = property on="2400_2_addr_superhyper" class="DigNum (strict)"() -> ("Value"=w5835:u8)  [unwired: 2 in, 2 out]
                    n4456 = Number To Fractional String(number=w5836) -> (F-format string=w5841:string)  [unwired: 3 in]
                    n4457 = Concatenate Strings(":INIT:IMM; :SOUR:CURR:LEV:IMM:AMPL " ("data"), w5841) -> (w5839:string)
                    n4458 = Number To Decimal String(number=w5835) -> (decimal integer string=w5837:string)  [unwired: 1 in]
                    n4459 = GPIB Write(0:w5837, 1:w5839, 2:i16 1 ("mode (0)")) -> ()  [unwired: 2 in, 2 out]
                  }
                  frame "2636_smua_SuperHyper" {
                    # "sweep voltage on 2636a smua"
                    n4460 = property on="SuperHyper" class="DigNum (strict)"() -> ("Value"=w5842:dbl)  [unwired: 2 in, 2 out]
                    n4461 = property on="Super_ministeps" class="DigNum (strict)"() -> ("Value"=w5843:dbl)  [unwired: 2 in, 2 out]
                    n4462 = property on="2336A_addr_superhyper" class="VISAName"() -> ("Value"=w5844:refnum<visa-resource-name>)  [unwired: 2 in, 2 out]
                    n4463 = Subtract(x=w5845, y=w5842) -> (x-y=w5846:dbl)
                    n4464 = Divide(x=w5846, y=w5843) -> (x/y=w5847:dbl)
                    n4465 = for {
                      N: w5843 -> [_]
                      tunnel: w5842 -> [w5857]
                      tunnel: w5847 -> [w5856]
                      tunnel: w5844 -> [w5853]
                      i -> [w5852]
                      n4466 = Increment(x=w5852) -> (x+1=w5851:i32)
                      n4467 = Multiply(x=w5856, y=w5851) -> (x*y=w5855:dbl)
                      n4468 = Add(x=w5855, y=w5857) -> (x+y=w5848:dbl)
                      n4469 = property on="diagona_super" class="Bool (strict)"() -> ("Value"=w5849:bool)  [unwired: 2 in, 2 out]
                      n4470 = call "setLevel.vi"("VISA resource name 2"=w5853, "Source"=Source."Voltage", "Channel"=Channel."a", "SourceLevel"=w5848) -> ("VISA resource name"=w5850:refnum<visa-resource-name>)  [unwired: 1 in, 2 out]
                      n4471 = Wait (ms)(milliseconds to wait=u32 12) -> ()  [unwired: 1 out]
                      n4472 = case shown="True" w5849 {
                        tunnel: w5848 -> [_ w5867]
                        tunnel: w5850 -> [_ w5862]
                        frame False {
                        }
                        frame True {
                          n4473 = property on="Slope_super" class="DigNum (strict)"() -> ("Value"=w5861:dbl)  [unwired: 2 in, 2 out]
                          n4474 = property on="Offset_super" class="DigNum (strict)"() -> ("Value"=w5860:dbl)  [unwired: 2 in, 2 out]
                          n4475 = Multiply(x=w5867, y=w5861) -> (x*y=w5866:dbl)
                          n4476 = Add(x=w5866, y=w5860) -> (x+y=w5863:dbl)
                          n4477 = call "setLevel.vi"("VISA resource name 2"=w5862, "Source"=Source."Voltage", "Channel"=Channel."b", "SourceLevel"=w5863) -> ()  [unwired: 1 in, 3 out]
                        }
                      }
                      n4478 = property on="SuperHyper" class="DigNum (strict)"("Value"=w5848) -> ()  [unwired: 2 in, 2 out]
                    }
                  }
                  frame "2636_smub_SuperHyper" {
                    # "sweep voltage on 2636a smua"
                    n4479 = property on="SuperHyper" class="DigNum (strict)"() -> ("Value"=w5868:dbl)  [unwired: 2 in, 2 out]
                    n4480 = property on="Super_ministeps" class="DigNum (strict)"() -> ("Value"=w5869:dbl)  [unwired: 2 in, 2 out]
                    n4481 = property on="2336A_addr_superhyper" class="VISAName"() -> ("Value"=w5870:refnum<visa-resource-name>)  [unwired: 2 in, 2 out]
                    n4482 = Subtract(x=w5871, y=w5868) -> (x-y=w5872:dbl)
                    n4483 = Divide(x=w5872, y=w5869) -> (x/y=w5873:dbl)
                    n4484 = for {
                      N: w5869 -> [_]
                      tunnel: w5868 -> [w5883]
                      tunnel: w5873 -> [w5882]
                      tunnel: w5870 -> [w5879]
                      i -> [w5878]
                      n4485 = Increment(x=w5878) -> (x+1=w5877:i32)
                      n4486 = Multiply(x=w5882, y=w5877) -> (x*y=w5881:dbl)
                      n4487 = Add(x=w5881, y=w5883) -> (x+y=w5874:dbl)
                      n4488 = property on="diagona_super" class="Bool (strict)"() -> ("Value"=w5875:bool)  [unwired: 2 in, 2 out]
                      n4489 = call "setLevel.vi"("VISA resource name 2"=w5879, "Source"=Source."Voltage", "Channel"=Channel."b", "SourceLevel"=w5874) -> ("VISA resource name"=w5876:refnum<visa-resource-name>)  [unwired: 1 in, 2 out]
                      n4490 = Wait (ms)(milliseconds to wait=u32 12) -> ()  [unwired: 1 out]
                      n4491 = case shown="True" w5875 {
                        tunnel: w5874 -> [_ w5893]
                        tunnel: w5876 -> [_ w5888]
                        frame False {
                        }
                        frame True {
